vi "Tusk.IsGlogalMessage.vi"(8 "error in (no error)":errorcluster, 10 "Message":string, 11 "Tusk in":refnum<class "Tusk.lvclass">) -> (0 "error out":errorcluster, 1 "Is Global Tusk Message?":bool, 3 "Tusk out":refnum<class "Tusk.lvclass">)   [LabVIEW 2018, in "Application.lvlib" / "Tusk.lvclass"]
uses:
  Tusk.lvclass
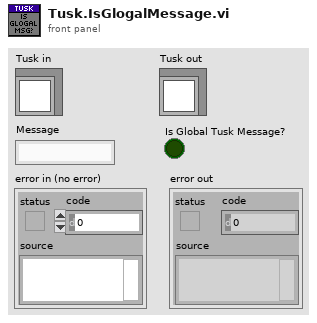
[diagram p1: front panel]
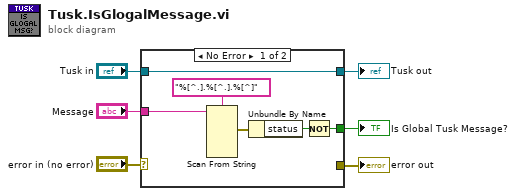
[diagram p0: block diagram]
diagram:
  n1 = case shown="No Error" "error in (no error)" {
    selector: "error in (no error)" -> [_ w14]
    tunnel: [_ w14] -> w5
    tunnel: [w12 w13] -> w3
    tunnel: "Tusk in" -> [w12 w13]
    tunnel: "Message" -> [w10 _]
    tunnel: [w7 _] -> w1
    frame No Error {
      n2 = Scan From String(format string="%[^.].%[^.].%[^]" ("regular expression"), input string=w10) -> (error out=w9:errorcluster)  [unwired: 8 in, 2 out]
      n3 = Unbundle By Name(w9) -> ("status"=w8:bool)
      n4 = Not(x=w8) -> (.not. x?=w7:bool)
    }
    frame Error {
    }
  }
  "error out" <- w5
  "Tusk out" <- w3
  "Is Global Tusk Message?" <- w1
